vi "836_CameraStart.vi"(8 "error in (no error)":errorcluster, 11 "CameraDevRef":T1) -> (0 "error out":errorcluster, 3 "CameraDevRef":T1)   [LabVIEW 2015]
doc: "Starts acquiring image data from the camera you specify. If an acquisition is already in progress, this VI increments the number of acquisition requests by one. After you start acquiring image data from the camera, you can use the Get Image VI in the FRC robot project to retrieve a specific image.\n\nThis software is licensed. Open the labview\\readme\\WPI Robotics Library Open Source License.txt file for more information."
uses:
  <vilib>/Rock Robotics/WPI/Camera/WPI_CameraDevRef.ctl
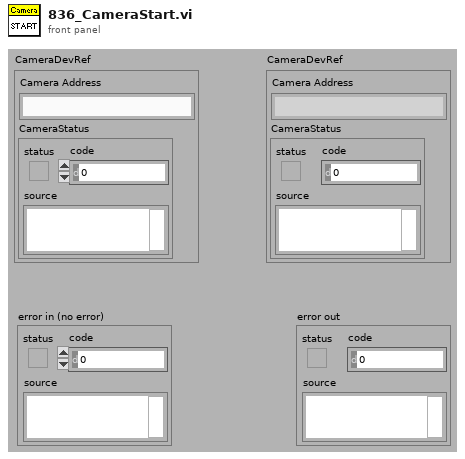
[diagram p1: front panel]
types:
  T1 = typedef "WPI_CameraDevRef.ctl" = cluster{"Camera Address":string, "CameraStatus":errorcluster}
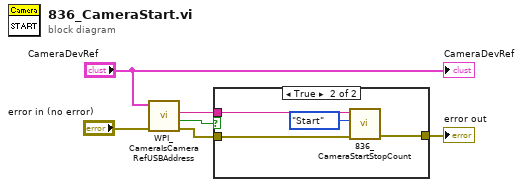
[diagram p0: block diagram]
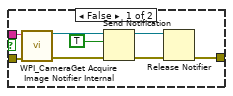
[diagram p2: hidden frame]
diagram:
  n1 = call <vilib>:"WPI_CameraIsCameraRefUSBAddress.vi"("error in (no error)"="error in (no error)", "CameraDevRef"="CameraDevRef") -> ("error out"=w5:errorcluster, "USB?"=w3:bool, "Camera Address Out"=w2:string)  [unwired: 6 in, 1 out]
  n2 = case shown="True" w3 {
    tunnel: [w11 w16] -> w6
    tunnel: w5 -> [w9 w17]
    tunnel: w2 -> [w8 w18]
    frame False {
      n3 = call <vilib>:"WPI_CameraGet Acquire Image Notifier Internal.vi"("error in (no error)"=w9, "Camera Address"=w8) -> ("error out"=w10:errorcluster, "Acquire Image Notifier"=w7:refnum<notifier>)  [unwired: 8 out]
      n4 = Send Notification(notification=TRUE, notifier=w7, error in (no error)=w10) -> (notifier out=w13:refnum<notifier>, error out=w12:errorcluster)
      n5 = Release Notifier(notifier=w13, error in (no error)=w12) -> (error out=w11:errorcluster)  [unwired: 3 out]
    }
    frame True {
      n6 = call <vilib>:"836_CameraStartStopCount.vi"("error in (no error)"=w17, "Action"=enum16{"Start", "Stop"}."Start", "Camera Address Out"=w18) -> ("error out"=w16:errorcluster)  [unwired: 8 in]
    }
  }
  "error out" <- w6
  "CameraDevRef" <- "CameraDevRef"
